vi "Handle.vi"(7 "Event Actor in":refnum<class "Event Actor.lvclass">, 11 "Nominal Event State in":refnum<class "Nominal Event State.lvclass">) -> (2 "Destroy?":bool, 5 "Event Actor out":refnum<class "Event Actor.lvclass">)   [LabVIEW 2021, in "jettl.lvlib" / "jettl Event Actor.lvlib" / "Nominal Event State.lvclass"]
uses:
  Nominal Event State.lvclass
  Actor/Event Actor/Event Actor.lvclass
  Nominal Event State.lvclass/Nominal Event State.ctl
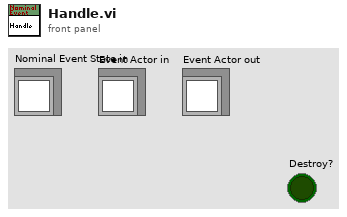
[diagram p1: front panel]
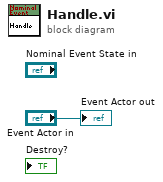
[diagram p0: block diagram]
diagram:
  "Event Actor out" <- "Event Actor in"
